vi "DemoT.vi"() -> ()   [LabVIEW 2018]
uses:
  RunningLog.lvclass
  RunningLog.lvclass/RunningLog.ctl
panel:
  in  "字符串":string="ASDGASDG ASDG ASDG SGD SDGASD"
  in  "路径":path=path "E:/#个人#/LabVIEW&C# Study/LVOOP2023YK/TESTFILE.txt"
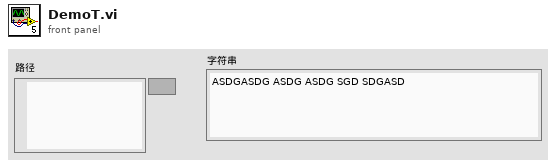
[diagram p1: front panel]
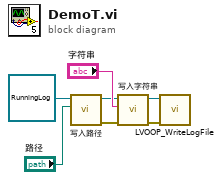
[diagram p0: block diagram]
diagram:
  n1 = call "写入路径.vi"("路径"="路径", "RunningLog输入"=refnum<class "RunningLog.lvclass"> refnum ("RunningLog.lvclass")) -> ("error out"=w4:errorcluster, "RunningLog输出"=w3:refnum<class "RunningLog.lvclass">)  [unwired: 8 in]
  n2 = call-dynamic "写入字符串.vi"("error in (no error)"=w4, "字符串"="字符串", "RunningLog输入"=w3) -> ("error out"=w1:errorcluster, "RunningLog输出"=w2:refnum<class "RunningLog.lvclass">)  [unwired: 7 in]
  n3 = call-dynamic "LVOOP_WriteLogFile.vi"("error in (no error)"=w1, "RunningLog 输入"=w2) -> ()  [unwired: 8 in, 2 out]
